vi "niFpgaTargetProperty_MergeVI.vi"   [LabVIEW 2017]
doc: "Gets or sets properties on an FPGA target in the Project Explorer window. The available properties depend on the FPGA target and some FPGA targets do not support any properties."
uses:
  <vilib>/eio/EIOPropertyNode/EIOPropertyNode.xnode
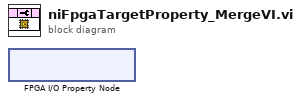
[diagram p0: block diagram]
diagram:
  n1 = xnode "FPGA I/O Property Node"() -> ()  [unwired: 1 in, 2 out]
